vi "Intake Control (SubVI).vi"(10 "Buttons":bool[](array[boolean]), 11 "Intake PID gains":T1={"proportional gain (Kc)"=0.9, "integral time (Ti, min)"=0.001, "derivative time (Td, min)"=0.0} {"derivative time (Td, min)" format="%.3f"; "integral time (Ti, min)" format="%.3f"; "proportional gain (Kc)" format="%.3f"}) -> ()   [LabVIEW 2014]
uses:
  <vilib>/Rock Robotics/WPI/Solenoid/WPI_SolenoidValue.ctl
  <vilib>/Rock Robotics/WPI/Solenoid/WPI_SolenoidSetEnum.vi
  <vilib>/addons/control/pid/pid.llb/PID (DBL).vi
  <vilib>/addons/control/pid/NI_PID_pid.lvlib
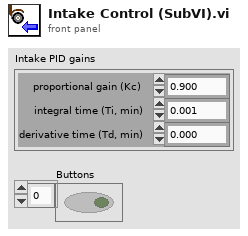
[diagram p1: front panel]
types:
  T1 = cluster{"proportional gain (Kc)":dbl, "integral time (Ti, min)":dbl, "derivative time (Td, min)":dbl}
  T2 = typedef "WPI_SolenoidValue.ctl" = enum16{"Off", "On", "Forward", "Reverse"}
  T3 = typedef "WPI_SwitchDevRef.ctl" = cluster{"DevStatus":errorcluster, "DIO Channel":T4, "Controller":T5, "CntIndex":T6, "Normally Closed":bool}
  T4 = typedef "FPGA_DIOChannel.ctl" = enum8{"DIO 0", "DIO 1", "DIO 2", "DIO 3", "DIO 4", "DIO 5", "DIO 6", "DIO 7", "DIO 8", "DIO 9", "DIO MXP 0", "DIO MXP 1", "DIO MXP 2", "DIO MXP 3", "DIO MXP 4", "DIO MXP 5", "DIO MXP 6", "DIO MXP 7", "DIO MXP 8", "DIO MXP 9", "DIO MXP 10", "DIO MXP 11", "DIO MXP 12", "DIO MXP 13", "DIO MXP 14", "DIO MXP 15", "Invalid"}
  T5 = typedef "FPGA_TypedefDigitalModule.ctl" = enum16{"Controller 1"}
  T6 = typedef "FPGA_CounterCtrSystemIndex.ctl" = enum8{"Ctr 0", "Ctr 1", "Ctr 2", "Ctr 3", "Ctr 4", "Ctr 5", "Ctr 6", "Ctr 7", "Invalid"}
  T7 = typedef "WPI_MotorControlDeviceRef.ctl" = cluster{"DeviceStatus":errorcluster, "Type":T8, "PWM":cluster{"Controller":T5, "PWM Channel":T9, "DeadBand":T10}, "CAN":cluster{"Device Number":u8, "Control Mode":T11, "Semaphore":T12, "Max Vout":dbl, "TalonSRX Control Mode":T13}, "Invert":bool, "TransformRef":T14, "InvTransformRef":T14}
  T8 = typedef "WPI_MotorControlType.ctl" = enum16{"PWM", "CAN", "CANTalonSRX"}
  T9 = typedef "FPGA_DIOPWMChannel.ctl" = enum8{"PWM 0", "PWM 1", "PWM 2", "PWM 3", "PWM 4", "PWM 5", "PWM 6", "PWM 7", "PWM 8", "PWM 9", "PWM MXP 0", "PWM MXP 1", "PWM MXP 2", "PWM MXP 3", "PWM MXP 4", "PWM MXP 5", "PWM MXP 6", "PWM MXP 7", "PWM MXP 8", "PWM MXP 9", "Invalid"}
  T10 = typedef "WPI_PWMDeadband.ctl" = cluster{"Name":string, "maxPositivePwm":i32, "minPositivePwm":i32, "centerPwm":i32, "maxNegativePwm":i32, "minNegativePwm":i32, "angularRange":u16}
  T11 = typedef "WPI_CANJaguar_ControlMode.ctl" = enum8{"Percent VBus", "Current", "Speed", "Position", "Voltage"}
  T12 = typedef "Semaphore RefNum" = refnum<k1>
  T13 = typedef "WPI_CANTalonSRX_APIControlMode.ctl" = enum8{"Percent VBus", "Speed", "Position", "Slave", "Unchanged / Invalid"}
  T14 = typedef "WPI_PWMTransform_ConPane.ctl" = refnum<vi>
  T15 = typedef "WPI_SolenoidDevRef.ctl" = cluster{"DevStatus":errorcluster, "Pneumatics Control Module":u8, "Forward Solenoid Channel":T16, "Reverse Solenoid Channel":T16}
  T16 = typedef "WPI_SolenoidChannel.ctl" = enum8{"Solenoid 0", "Solenoid 1", "Solenoid 2", "Solenoid 3", "Solenoid 4", "Solenoid 5", "Solenoid 6", "Solenoid 7", "Invalid"}
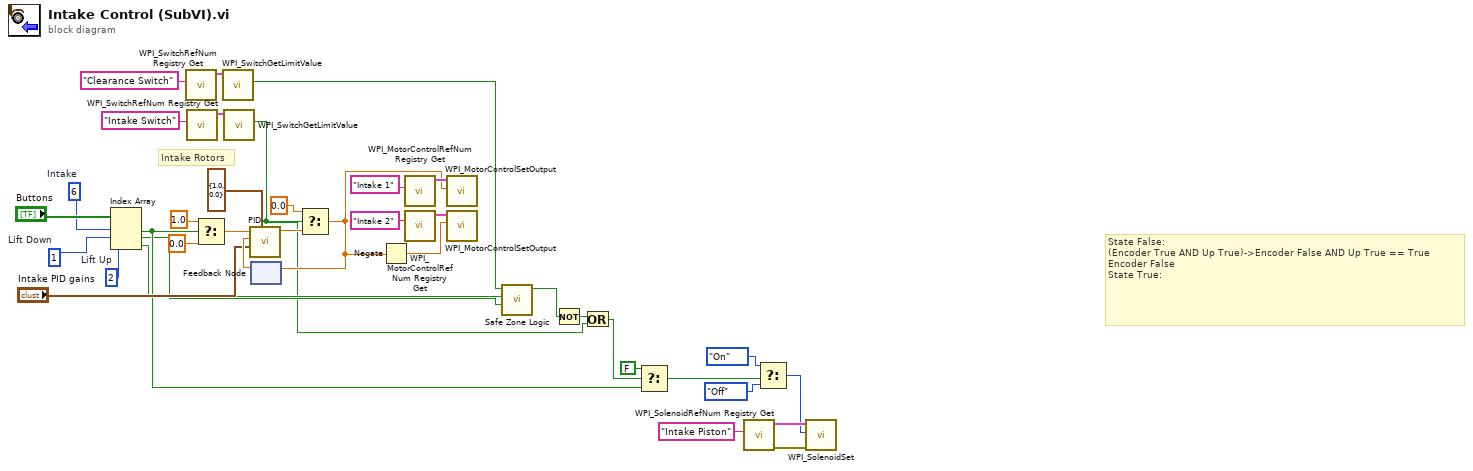
[diagram p0: block diagram]
diagram:
  w8 = 2  # Lift Up
  w9 = 1  # Lift Down
  w37 = 6  # Intake
  # "State False:\n(Encoder True AND Up True)->Encoder False AND Up True == True\nEncoder False\nState True:"
  # "Intake Rotors"
  n1 = Index Array(array="Buttons", index #1=w37, index #2=w9, index #3=w8) -> (element #1=w13:bool, element #2=w5:bool, element #3=w6:bool)
  n2 = call <vilib>:"WPI_SwitchRefNum Registry Get.vi"("refnum name"="Clearance Switch") -> ("SwitchDevRef"=w10:T3)  [unwired: 9 in, 1 out]
  n3 = call <vilib>:"WPI_SwitchRefNum Registry Get.vi"("refnum name"="Intake Switch") -> ("SwitchDevRef"=w19:T3)  [unwired: 9 in, 1 out]
  n4 = Select(t=1.0 ("setpoint"), s=w13, f=0.0) -> (s? t:f=w36:dbl)
  n5 = call <vilib>:"WPI_SwitchGetLimitValue.vi"("SwitchDevRef"=w10) -> ("Switch Pressed"=w7:bool)  [unwired: 8 in, 2 out]
  n6 = call <vilib>:"WPI_SwitchGetLimitValue.vi"("SwitchDevRef"=w19) -> ("Switch Pressed"=w2:bool)  [unwired: 8 in, 2 out]
  n7 = feedback #1() -> (w33:dbl)  [unwired: 1 in]
  n8 = call-poly <vilib>:"PID.vi"("output range"=cluster{"output high":dbl, "output low":dbl} {"output high"=1.0, "output low"=0.0}, "PID gains"="Intake PID gains", "process variable"=w33, "setpoint"=w36) -> ("output"=w17:dbl)  [unwired: 6 in, 1 out]
  n9 = Select(t=0.0, s=w2, f=w17) -> (s? t:f=w16:dbl)
  n10 = feedback-in #1(w16) -> ()
  n11 = Negate(x=w16) -> (-x=w34:dbl)
  n12 = call <vilib>:"WPI_MotorControlRefNum Registry Get.vi"("refnum name"="Intake 1") -> ("MotorControlDevRef"=w27:T7)  [unwired: 9 in, 1 out]
  n13 = call <vilib>:"WPI_MotorControlRefNum Registry Get.vi"("refnum name"="Intake 2") -> ("MotorControlDevRef"=w28:T7)  [unwired: 9 in, 1 out]
  n14 = call <vilib>:"WPI_MotorControlSetOutput.vi"("Output"=w16, "MotorControlDevRef"=w27) -> ()  [unwired: 7 in, 3 out]
  n15 = call <vilib>:"WPI_MotorControlSetOutput.vi"("Output"=w34, "MotorControlDevRef"=w28) -> ()  [unwired: 7 in, 3 out]
  n16 = call "Safe Zone Logic.vi"("Down"=w5, "Up"=w6, "Limit Switch"=w7) -> ("Safe Zone"=w4:bool)  [unwired: 8 in]
  n17 = Not(x=w4) -> (.not. x?=w3:bool)
  n18 = Or(x=w3, y=w2) -> (x .or. y?=w1:bool)
  n19 = Select(t=FALSE, s=w1, f=w13) -> (s? t:f=w14:bool)
  n20 = call <vilib>:"WPI_SolenoidRefNum Registry Get.vi"("refnum name"="Intake Piston") -> ("error out"=w25:errorcluster, "SolenoidDevRef"=w24:T15)  [unwired: 9 in]
  n21 = Select(t=WPI_SolenoidValue."On" ("Value"), s=w14, f=WPI_SolenoidValue."Off" ("Value")) -> (s? t:f=w21:T2)
  n22 = call-poly <vilib>:"WPI_SolenoidSet.vi"("error in (no error)"=w25, "Value"=w21, "SolenoidDevRef"=w24) -> ()  [unwired: 7 in, 2 out]
